vi "VPSW Vapor Pressure of Saline Water Raoult's Formula (Pa).vi"(1 "Salinity":dbl, 2 "Tceg":dbl[unit]) -> (0 "VPSW":dbl[unit])   [LabVIEW 2018]
panel:
  out "VPPW":dbl[unit]
  out "Temprature of Pure Water \nKelvin Degree":dbl[unit](slide) scale=273.0..373.0
  out "Tk":dbl[unit]
  out "Temprature of Pure Water\nCentigrade Degree":dbl[unit](slide) scale=0.0..100.0
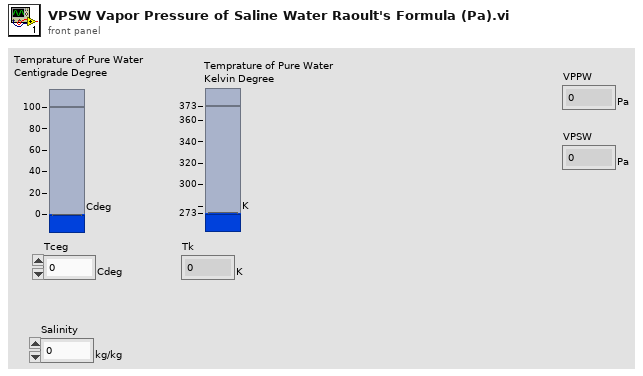
[diagram p1: front panel]
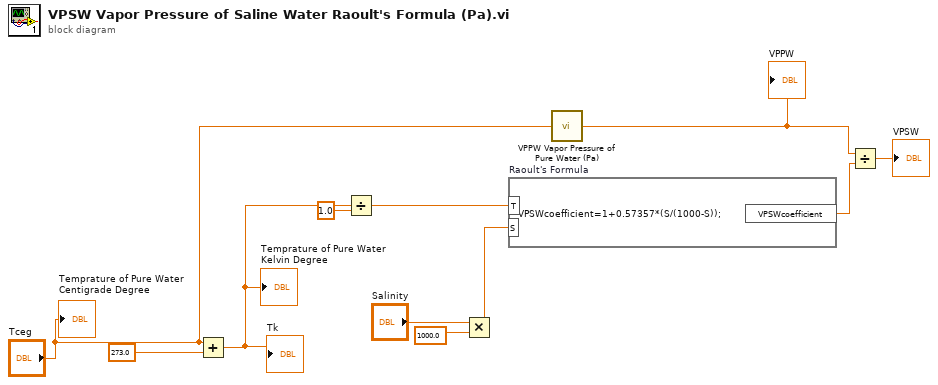
[diagram p0: block diagram]
diagram:
  n1 = Add(x="Tceg", y=dbl[unit] 273.0) -> (x+y=w8:dbl[unit])
  "Tk" <- w8
  "Temprature of Pure Water \nKelvin Degree" <- w8
  n2 = Divide(x=w8, y=dbl[unit] 1.0) -> (x/y=w11:dbl)
  n3 = Multiply(x="Salinity", y=1000.0) -> (x*y=w2:dbl)
  n4 = formula code="VPSWcoefficient=1+0.57357*(S/(1000-S));" "Raoult's Formula"("T"=w11, "S"=w2) -> ("VPSWcoefficient"=w6:dbl)
  n5 = call "VPPW Vapor Pressure of Pure Water (Pa).vi"("Tceg"="Tceg") -> ("VPPW"=w7:dbl[unit])
  "VPPW" <- w7
  n6 = Divide(x=w7, y=w6) -> (x/y=→"VPSW":dbl[unit])
  "Temprature of Pure Water\nCentigrade Degree" <- "Tceg"
